vi "Test Get VIs.vi"(8 "Error In":errorcluster) -> ()   [LabVIEW 2014]
uses:
  <vilib>/Utility/traverseref.llb/TRef TravTarget.ctl
  <vilib>/Utility/traverseref.llb/VI Scripting - Traverse.lvlib
panel:
  out "Wires and connected ClassNames in for loop.":string[][](array[string])
  out "Objects[] in for loop":string[](array[string])
  out "All Objects[]":string[](array[string])
  in  "vi path":path
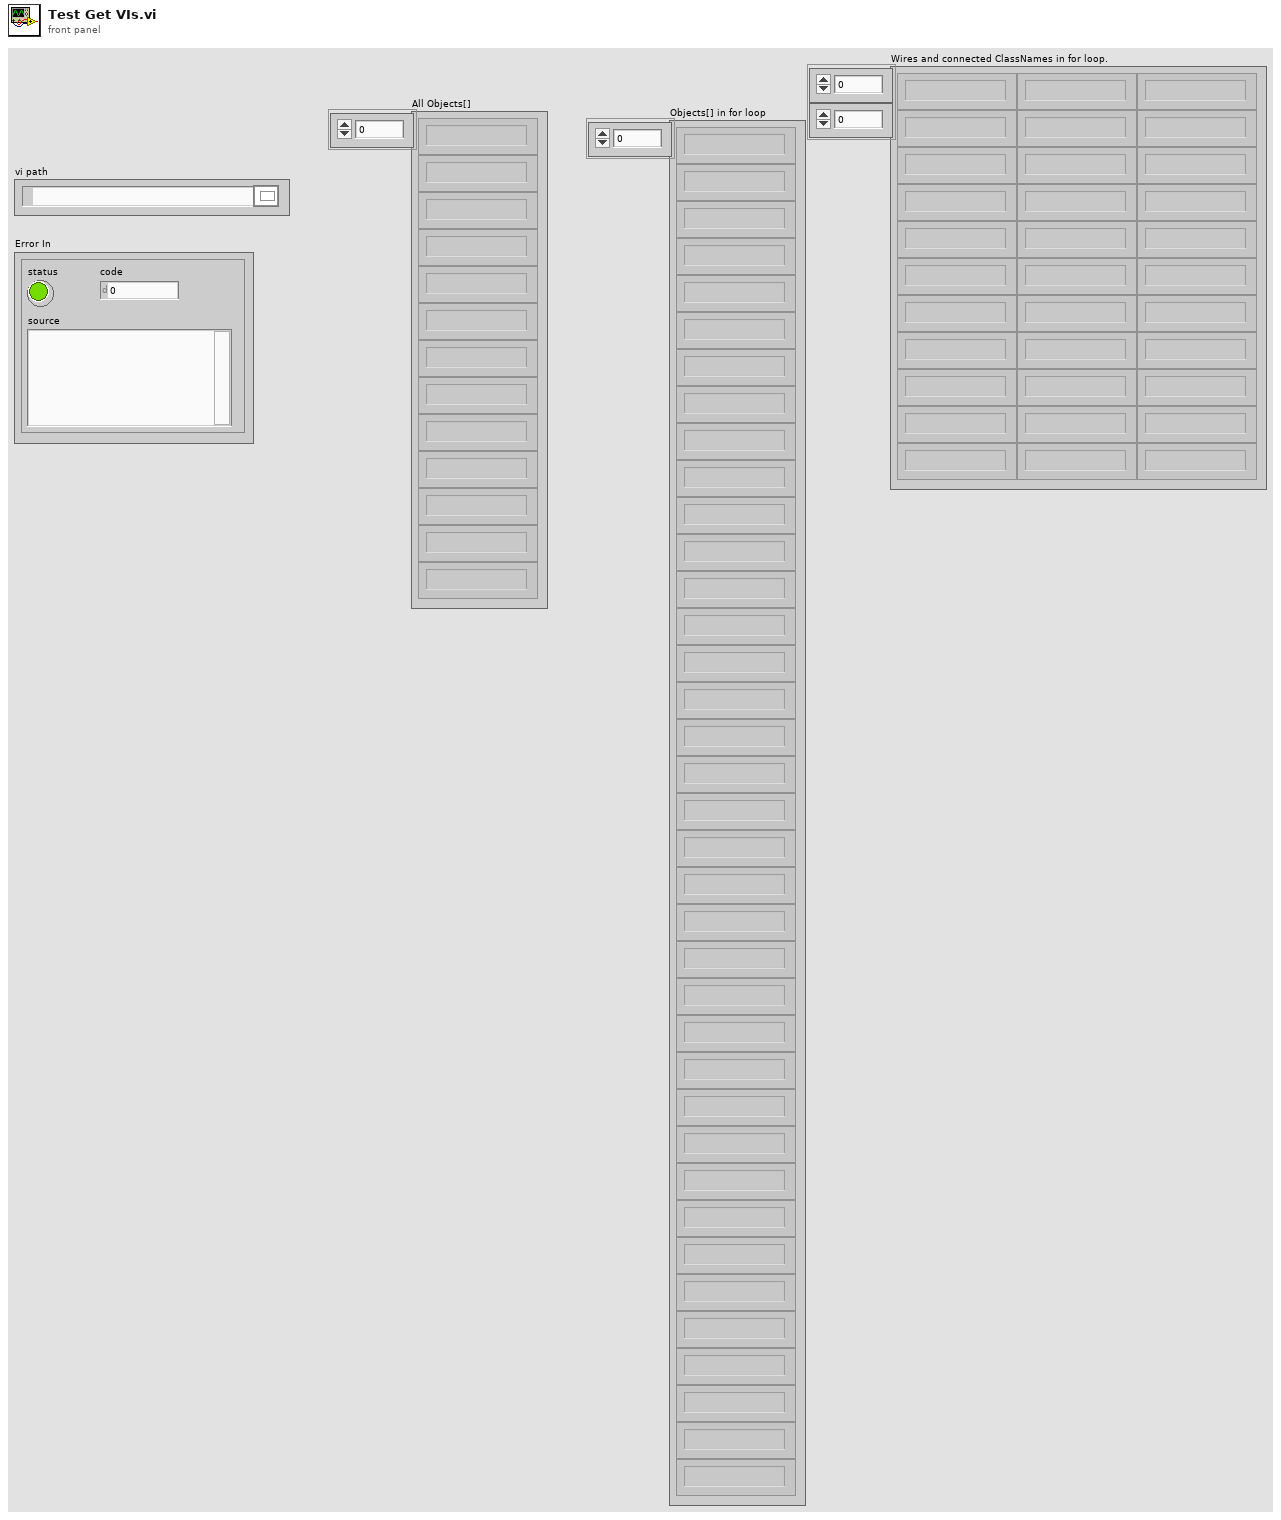
[diagram p1: front panel]
types:
  T1 = typedef "TRef TravTarget.ctl" = enum16{"FP", "BD", "Other"}
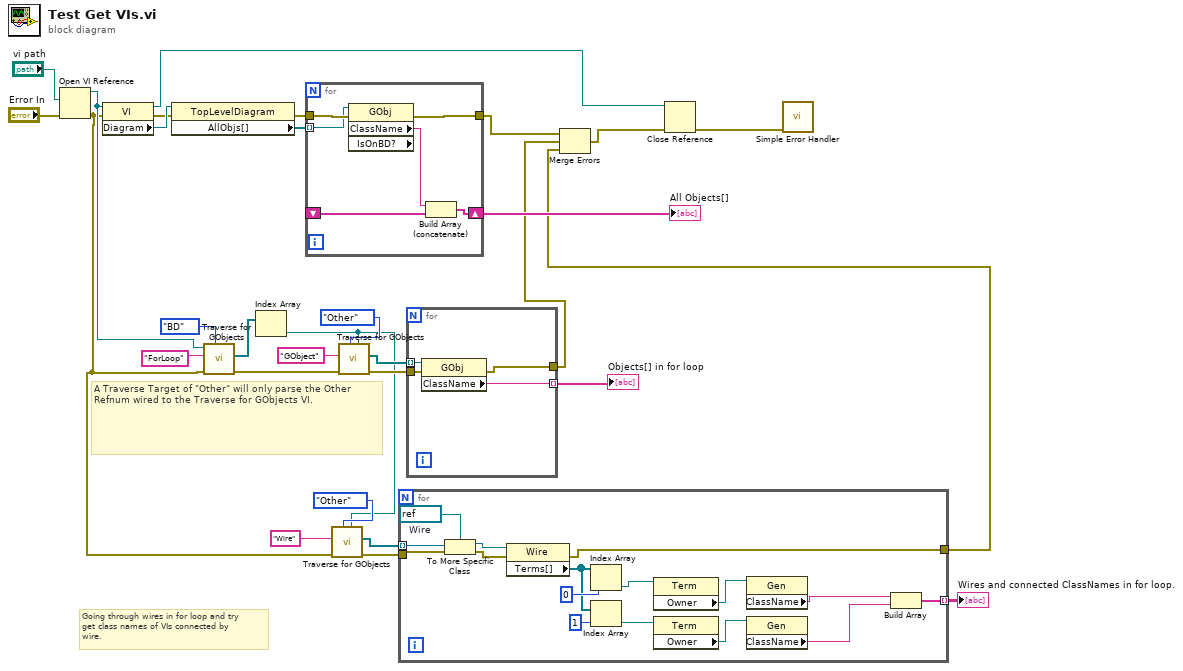
[diagram p0: block diagram]
diagram:
  # "Going through wires in for loop and try\nget class names of VIs connected by\nwire."
  # "A Traverse Target of \"Other\" will only parse the Other Refnum wired to the Traverse for GObjects VI."
  n1 = Open VI Reference(vi path="vi path", error in (no error)="Error In") -> (vi reference=w16:refnum<vi>, error out=w3:errorcluster)  [unwired: 4 in]
  n2 = property class="VI"(reference=w16, error in=w3) -> (reference out=w28:refnum<vi>, error out=w26:errorcluster, "Diagram"=w27:refnum<vi>)
  n3 = property class="TopLevelDiagram"(reference=w27, error in=w26) -> (error out=w24:errorcluster, "AllObjs[]"=w23:refnum<vi>[])  [unwired: 1 out]
  n4 = call <vilib>:"Traverse for GObjects.vi"("Traverse Target"=TRef_TravTarget."BD", "error in (no error)"=w3, "Class Name"="ForLoop", "VI Refnum"=w16) -> ("error out"=w19:errorcluster, "References"=w20:refnum<vi>[])  [unwired: 4 in, 2 out]
  n5 = Index Array(array=w20) -> (element=w4:refnum<vi>)  [unwired: 1 in]
  n6 = for {
    tunnel: w24 -> [w36]
    tunnel: w23 -> [w35] mode=indexing
    shift-right: [w32] -> w22
    shift-left: _ -> [w33]
    tunnel: [w31] -> w11
    n7 = property class="GObj" props=["ClassName", "IsOnBD?"](reference=w35, error in=w36) -> (error out=w31:errorcluster, "ClassName"=w34:string)  [unwired: 2 out]
    n8 = Build Array (concatenate)(w34, w33) -> (w32:string[])
  }
  "All Objects[]" <- w22
  n9 = call <vilib>:"Traverse for GObjects.vi"("Other Refnum"=w4, "Traverse Target"=TRef_TravTarget."Other", "error in (no error)"=w3, "Class Name"="Wire") -> ("error out"=w7:errorcluster, "References"=w8:refnum<vi>[])  [unwired: 4 in, 2 out]
  n10 = call <vilib>:"Traverse for GObjects.vi"("Other Refnum"=w4, "Traverse Target"=TRef_TravTarget."Other", "error in (no error)"=w19, "Class Name"="GObject") -> ("error out"=w14:errorcluster, "References"=w13:refnum<vi>[])  [unwired: 4 in, 2 out]
  n11 = for {
    tunnel: w7 -> [w50]
    tunnel: w8 -> [w51] mode=indexing
    tunnel: [w52] -> w2
    tunnel: [w42] -> w1 mode=indexing
    w49 = refnum<vi> refnum  # Wire
    n12 = To More Specific Class(target class=w49, reference=w51, error in=w50) -> (specific class reference=w48:refnum<vi>, error out=w47:errorcluster)
    n13 = property class="Wire"(reference=w48, error in=w47) -> (error out=w52:errorcluster, "Terms[]"=w37:refnum<vi>[])  [unwired: 1 out]
    n14 = Index Array(array=w37, index=0) -> (element=w44:refnum<vi>)
    n15 = Index Array(array=w37, index=1) -> (element=w43:refnum<vi>)
    n16 = property class="Term"(reference=w44) -> ("Owner"=w41:refnum<vi>)  [unwired: 1 in, 2 out]
    n17 = property class="Term"(reference=w43) -> ("Owner"=w40:refnum<vi>)  [unwired: 1 in, 2 out]
    n18 = property class="Gen"(reference=w41) -> ("ClassName"=w38:string)  [unwired: 1 in, 2 out]
    n19 = property class="Gen"(reference=w40) -> ("ClassName"=w39:string)  [unwired: 1 in, 2 out]
    n20 = Build Array(w38, w39) -> (w42:string[])
  }
  "Wires and connected ClassNames in for loop." <- w1
  n21 = for {
    tunnel: w14 -> [w56]
    tunnel: w13 -> [w55] mode=indexing
    tunnel: [w54] -> w12 mode=indexing
    tunnel: [w53] -> w10
    n22 = property class="GObj"(reference=w55, error in=w56) -> (error out=w53:errorcluster, "ClassName"=w54:string)  [unwired: 1 out]
  }
  "Objects[] in for loop" <- w12
  n23 = Merge Errors(w11, w10, w2) -> (w9:errorcluster)
  n24 = Close Reference(reference=w28, error in (no error)=w9) -> (error out=w29:errorcluster)
  n25 = call <vilib>:"Simple Error Handler.vi"("error in (no error)"=w29) -> ()  [unwired: 4 in, 5 out]
